vi "Communication Information.vi"(8 "Total Interrupt":i32, 9 "Total Error Answer":i32, 10 "Total Answer":i32, 11 "Total Request":i32) -> (3 "output array":string[][](array[string]))   [LabVIEW 2020, in "ModBus Serial Master.lvlib"]
uses:
  ModBus Serial Master.lvlib
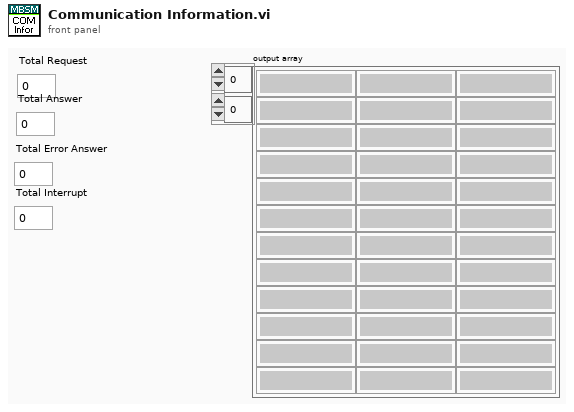
[diagram p1: front panel]
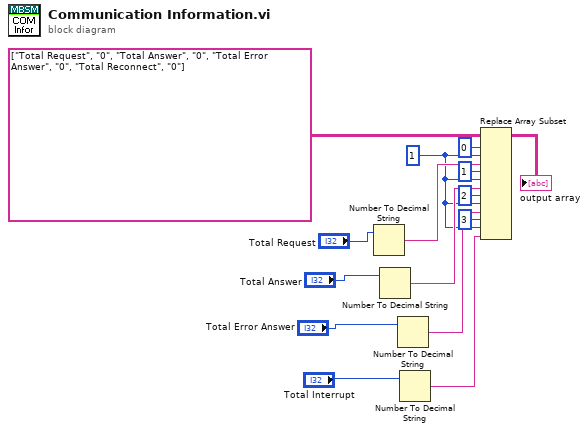
[diagram p0: block diagram]
diagram:
  w5 = 1 ("disabled index (col)")
  n1 = Number To Decimal String(number="Total Request") -> (decimal integer string=w12:string)  [unwired: 1 in]
  n2 = Number To Decimal String(number="Total Answer") -> (decimal integer string=w9:string)  [unwired: 1 in]
  n3 = Number To Decimal String(number="Total Error Answer") -> (decimal integer string=w7:string)  [unwired: 1 in]
  n4 = Number To Decimal String(number="Total Interrupt") -> (decimal integer string=w3:string)  [unwired: 1 in]
  n5 = Replace Array Subset(array=string[][] [["Total Request", "0"], ["Total Answer", "0"], ["Total Error Answer", "0"], ["Total Reconnect", "0"]], new element #1=w12, index (row) #1=0 ("disabled index (row)"), index (col) #1=w5, new element #2=w9, index (row) #2=1 ("disabled index (row)"), index (col) #2=w5, new element #3=w7, index (row) #3=2 ("disabled index (row)"), index (col) #3=w5, new element #4=w3, index (row) #4=3 ("disabled index (row)"), index (col) #4=w5) -> (→"output array":string[][])
